vi "FITS hdr gen row int.vi"(5 "Format":string, 9 "Comment":string, 10 "Value":i32, 11 "Field":string) -> (3 "FITS Row":string)   [LabVIEW 2024]
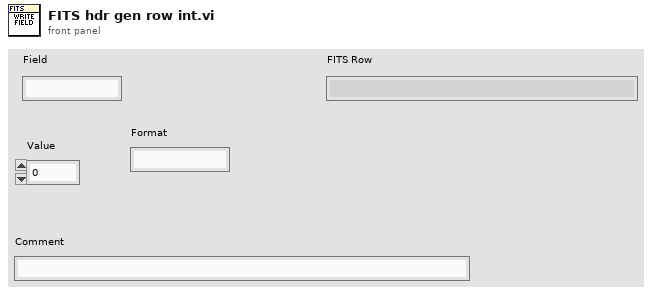
[diagram p1: front panel]
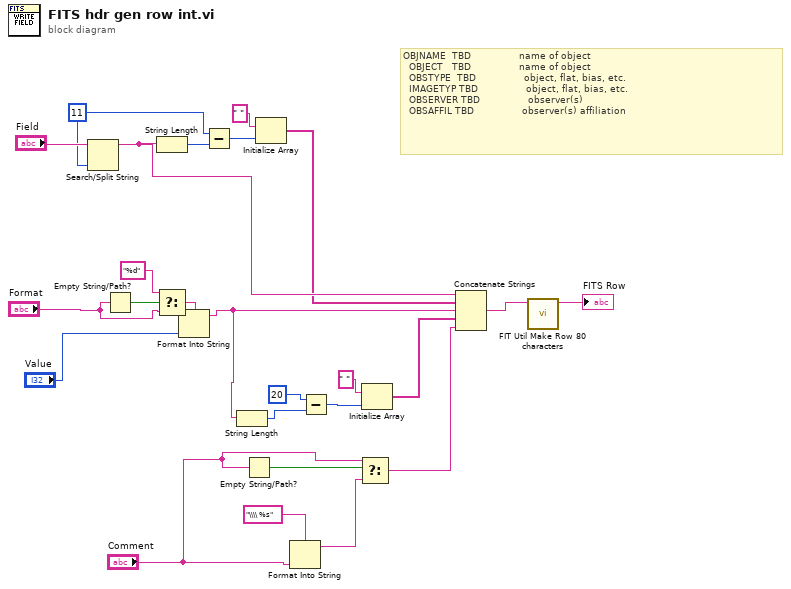
[diagram p0: block diagram]
diagram:
  w24 = 11
  # "OBJNAME  TBD                name of object\n  OBJECT   TBD                name of object\n  OBSTYPE  TBD                object, flat, bias, etc.\n  IMAGETYP TBD                object, flat, bias, etc.\n  OBSERVER TBD                observer(s) \n  OBSAFFIL TBD                observer(s) affiliation"
  n1 = Search/Split String(string="Field", offset (0)=w24) -> (substring before match=w17:string)  [unwired: 1 in, 2 out]
  n2 = Empty String/Path?(string/path="Format") -> (empty?=w14:bool)
  n3 = String Length(string=w17) -> (length=w23:i32)
  n4 = Select(t="%d", s=w14, f="Format") -> (s? t:f=w12:string)
  n5 = Format Into String(format string=w12, "Value") -> (resulting string=w6:string)  [unwired: 2 in, 1 out]
  n6 = Subtract(x=w24, y=w23) -> (x-y=w22:i32)
  n7 = String Length(string=w6) -> (length=w8:i32)
  n8 = Empty String/Path?(string/path="Comment") -> (empty?=w4:bool)
  n9 = Initialize Array(" ", w22) -> (w16:string[])
  n10 = Format Into String(format string="\\\\ %s", "Comment") -> (resulting string=w2:string)  [unwired: 2 in, 1 out]
  n11 = Subtract(x=20, y=w8) -> (x-y=w7:i32)
  n12 = Select(t="Comment", s=w4, f=w2) -> (s? t:f=w1:string)
  n13 = Initialize Array(" ", w7) -> (w5:string[])
  n14 = Concatenate Strings(w17, w16, w6, w5, w1) -> (w15:string)
  n15 = call "FIT Util Make Row 80 characters.vi"("Row"=w15) -> ("Row with 80 char"=→"FITS Row":string)  [unwired: 10 in]
